vi "SP_DORG.vi"(3 "Commands":string[](array[string])) -> (1 "Commands Out":string[](array[string]))   [LabVIEW 2009]
panel:
  # "This LabVIEW item is deprecated.\n\nIt is believed to be unused and will be removed in a future version of SRV."
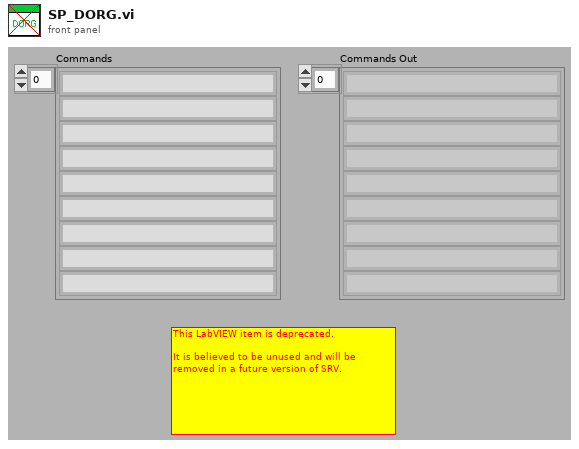
[diagram p1: front panel]
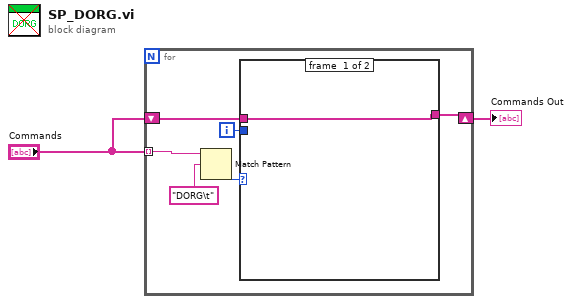
[diagram p0: block diagram]
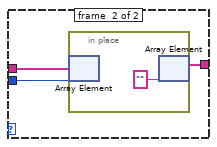
[diagram p2: hidden frame]
diagram:
  n1 = for {
    tunnel: "Commands" -> [w6] mode=indexing
    shift-right: [w3] -> w1
    shift-left: "Commands" -> [w5]
    i -> [w4]
    n2 = Match Pattern(string=w6, regular expression="DORG\t") -> (offset past match=w7:i32)  [unwired: 1 in, 3 out]
    n3 = case shown="Default" w7 {
      tunnel: w5 -> [w9 w12]
      tunnel: w4 -> [_ w11]
      tunnel: [w9 w10] -> w3
      frame #0 {
      }
      frame #1 {
        n4 = in-place {
          n5 = in-place-array #1(w12, w11) -> ()  [unwired: 1 out]
          n6 = in-place-array #1("" ("regular expression")) -> (w10:string[])  [unwired: 1 out]
        }
      }
    }
  }
  "Commands Out" <- w1
